vi "SpectrumDeltaE.vi"(3 "Select DeltaE":enum16{"Delta E 2000", "CMC 1:1 ", "CMC 2:1"}(ring), 4 "Iluminant - RGB - CMF":T2, 5 "Reflectance 2":dbl[](array[numeric]), 6 "Reflectance 1":dbl[](array[numeric])) -> (0 "Color1":T1, 1 "Delta E":dbl, 2 "Color2":T1)   [LabVIEW 2013]
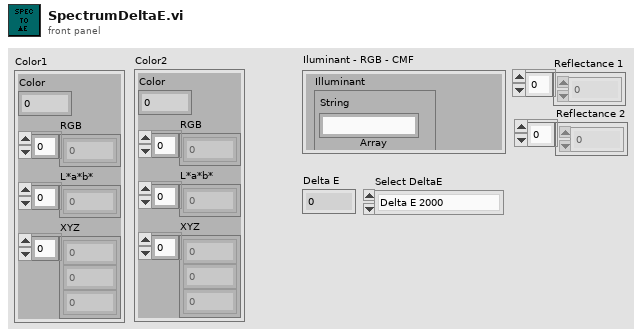
[diagram p1: front panel]
types:
  T1 = cluster{"Color":u32, "RGB":dbl[], "L*a*b*":dbl[], "XYZ":dbl[]}
  T2 = cluster{"Illuminant":cluster{"String":string, "Array":dbl[]}, "Selected RGB":string, "CMF":dbl[][]}
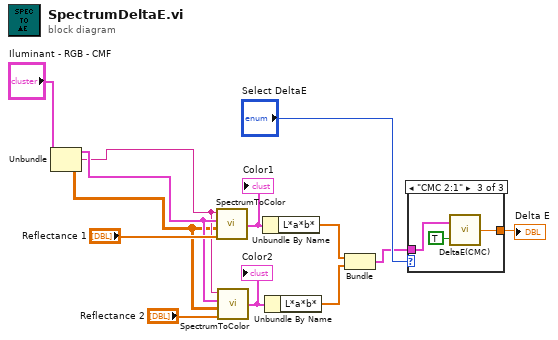
[diagram p0: block diagram]
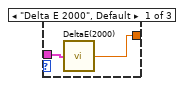
[diagram p2: hidden frame]
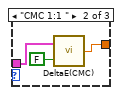
[diagram p3: hidden frame]
diagram:
  n1 = Unbundle("Iluminant - RGB - CMF") -> ("Illuminant"=w3:cluster{"String":string, "Array":dbl[]}, "Selected RGB"=w2:string, "CMF"=w1:dbl[][])
  n2 = call "SpectrumToColor.vi"("Reflectance"="Reflectance 1", "CMF"=w1, "Illuminant"=w3, "Selected RGB"=w2) -> ("Color,XYZ,RGB,Lab"=w11:T1)
  "Color1" <- w11
  n3 = call "SpectrumToColor.vi"("Reflectance"="Reflectance 2", "CMF"=w1, "Illuminant"=w3, "Selected RGB"=w2) -> ("Color,XYZ,RGB,Lab"=w10:T1)
  "Color2" <- w10
  n4 = Unbundle By Name(w11) -> ("L*a*b*"=w8:dbl[])
  n5 = Unbundle By Name(w10) -> ("L*a*b*"=w7:dbl[])
  n6 = Bundle("L*a*b*"=w8, "L*a*b*"=w7) -> (w6:cluster{"L*a*b*":dbl[], "L*a*b*":dbl[]})  [unwired: 1 in]
  n7 = case shown="\"CMC 2:1\"" "Select DeltaE" {
    tunnel: w6 -> [w15 w18 w21]
    tunnel: [w14 w16 w19] -> w5
    frame "Delta E 2000", Default {
      n8 = call "DeltaE(2000).vi"("L*a*b Colors"=w15) -> ("Delta E"=w14:dbl)
    }
    frame "CMC 1:1 " {
      n9 = call "DeltaE(CMC).vi"("l:c"=FALSE, "L*a*b colors"=w18) -> ("Delta E"=w16:dbl)
    }
    frame "CMC 2:1" {
      n10 = call "DeltaE(CMC).vi"("l:c"=TRUE, "L*a*b colors"=w21) -> ("Delta E"=w19:dbl)
    }
  }
  "Delta E" <- w5
